vi "CAN Signal to Data.vi"(8 "Fehler (Eingang, kein Fehler)":errorcluster, 9 "PayldLen":u32, 10 "payload":u8[](array[numeric]), 11 "Referenz (Eingang)":refnum<k21>) -> (0 "Fehler (Ausgang)":errorcluster, 2 "NameShort":string, 3 "value":dbl)   [LabVIEW 2020]
uses:
  <resource>/objmgr/xnet.rc
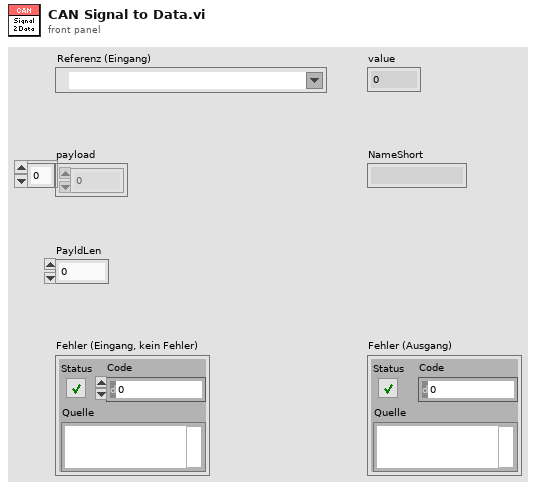
[diagram p1: front panel]
types:
  T1 = cluster{"Start Byte":i32, "Byte Length":i32, "Byte Order":enum16{"Motorola", "Intel"}, "Data Type":enum16{"Unsigned", "Signed", "Float"}, "Scale Factor":dbl, "Scale Offset":dbl}
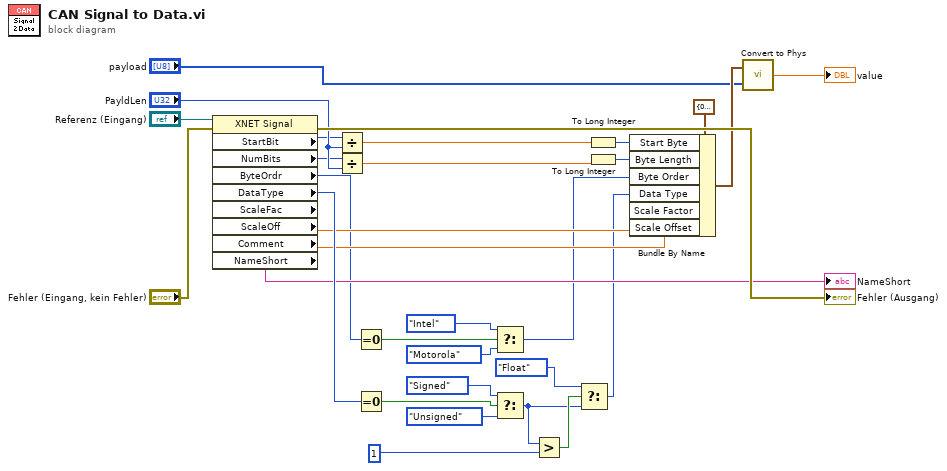
[diagram p0: block diagram]
diagram:
  n1 = property class="XNET Signal" props=["StartBit", "NumBits", "ByteOrdr", "DataType", "ScaleFac", "ScaleOff", "Comment", "NameShort"](reference="Referenz (Eingang)", error in="Fehler (Eingang, kein Fehler)") -> (error out=→"Fehler (Ausgang)":errorcluster, "StartBit"=w13:u32, "NumBits"=w14:u32, "ByteOrdr"=w9:u32, "DataType"=w31:u32, "ScaleFac"=w15:dbl, "ScaleOff"=w16:dbl, "NameShort"=→"NameShort":string)  [unwired: 2 out]
  n2 = Divide(x=w13, y="PayldLen") -> (x/y=w19:dbl)
  n3 = Divide(x=w14, y="PayldLen") -> (x/y=w20:dbl)
  n4 = Equal To 0?(x=w9) -> (x = 0?=w10:bool)
  n5 = Equal To 0?(x=w31) -> (x = 0?=w30:bool)
  n6 = Select(t=enum16{"Motorola", "Intel"}."Intel" ("Byte Order"), s=w10, f=enum16{"Motorola", "Intel"}."Motorola" ("Byte Order")) -> (s? t:f=w8:enum16{"Motorola", "Intel"})
  n7 = Select(t=enum16{"Unsigned", "Signed", "Float"}."Signed" ("Data Type"), s=w30, f=enum16{"Unsigned", "Signed", "Float"}."Unsigned" ("Data Type")) -> (s? t:f=w2:enum16{"Unsigned", "Signed", "Float"})
  n8 = Greater?(x=w2, y=u32 1 ("PayldLen")) -> (0:w3:bool)
  n9 = Select(t=enum16{"Unsigned", "Signed", "Float"}."Float" ("s? t:f"), s=w3, f=w2) -> (s? t:f=w5:enum16{"Unsigned", "Signed", "Float"})
  n10 = To Long Integer(number=w19) -> (32bit integer=w26:i32)
  n11 = To Long Integer(number=w20) -> (32bit integer=w27:i32)
  n12 = Bundle By Name(cluster=T1 {"Start Byte"=0, "Byte Length"=0, "Byte Order"=enum."Motorola", "Data Type"=enum."Unsigned", "Scale Factor"=0.0, "Scale Offset"=0.0} ("type descriptor"), "Start Byte"=w26, "Byte Length"=w27, "Byte Order"=w8, "Data Type"=w5, "Scale Factor"=w15, "Scale Offset"=w16) -> (w17:T1)
  n13 = call <vilib>:"Convert to Phys.vi"("data in"="payload", "type descriptor"=w17) -> ("value"=→"value":dbl)
